vi "Remove Empty Strings.vi"(0 "instrument types in":string[](array[string])) -> (4 "instrument types out":string[](array[string]))   [LabVIEW 2021, in "Converter.lvlib"]
uses:
  Converter.lvlib
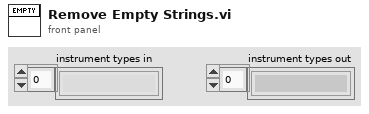
[diagram p1: front panel]
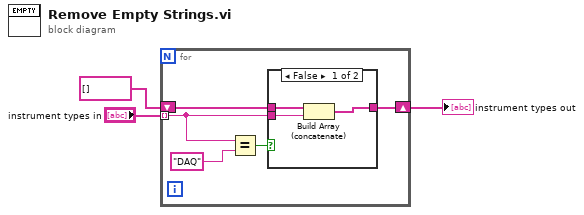
[diagram p0: block diagram]
diagram:
  n1 = for {
    tunnel: "instrument types in" -> [w4] mode=indexing
    shift-right: [w7] -> w3
    shift-left: string[] [] -> [w6]
    n2 = Equal?(x=w4, y="DAQ") -> (x = y?=w8:bool)
    n3 = case shown="False" w8 {
      tunnel: [w9 w12] -> w7
      tunnel: w6 -> [w10 w12]
      tunnel: w4 -> [w11 _]
      frame False {
        n4 = Build Array (concatenate)(w10, w11) -> (w9:string[])
      }
      frame True {
      }
    }
  }
  "instrument types out" <- w3
